vi "sendqueue.vi"   [LabVIEW 2025]
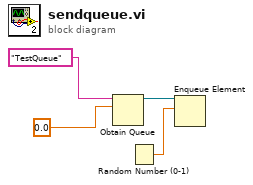
[diagram p0: block diagram]
diagram:
  n1 = Obtain Queue(name (unnamed)="TestQueue", element data type=0.0) -> (queue out=w2:refnum<queue>)  [unwired: 3 in, 2 out]
  n2 = Random Number (0-1)() -> (number: 0 to 1=w1:dbl)
  n3 = Enqueue Element(queue=w2, element=w1) -> ()  [unwired: 2 in, 3 out]
